vi "Delete Process.vi"(8 "Error In":errorcluster, 10 "Process Name":string, 11 "CS++DSCManager in":refnum<class "CS++DSCManager.lvclass">) -> (0 "Error Out":errorcluster, 3 "CS++DSCManager out":refnum<class "CS++DSCManager.lvclass">)   [LabVIEW 2016, in "CS++DSCManager.lvlib" / "CS++DSCManager.lvclass"]
doc: "Removes a process and its associated variables from the Shared Variable Engine (SVE)."
uses:
  CS++DSCManager.lvclass
  <vilib>/lvdsc/NI_DSC.lvlib
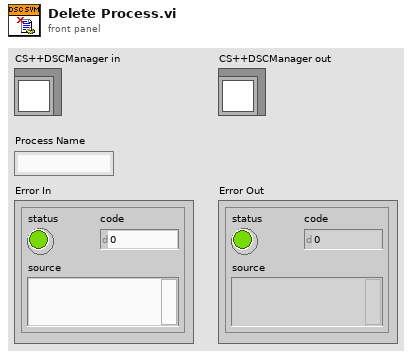
[diagram p1: front panel]
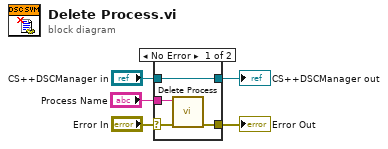
[diagram p0: block diagram]
diagram:
  n1 = case shown="No Error" "Error In" {
    selector: "Error In" -> [w7 w11]
    tunnel: [w6 w11] -> w4
    tunnel: [w9 w10] -> w2
    tunnel: "CS++DSCManager in" -> [w9 w10]
    tunnel: "Process Name" -> [w8 _]
    frame No Error {
      n2 = call <vilib>:"Delete Process.vi"("error in (no error)"=w7, "process name"=w8) -> ("error out"=w6:errorcluster)  [unwired: 9 in]
    }
    frame Error {
    }
  }
  "Error Out" <- w4
  "CS++DSCManager out" <- w2
